vi "measVoltHzOffset.vi"() -> (1 "Error":bool)   [LabVIEW 2014]
uses:
  <vilib>/Platform/TimedLoop/XDataNode/timing_clust.ctl
  <vilib>/Platform/TimedLoop/XDataNode/nitl_modes.ctl
  <vilib>/Platform/TimedLoop/XDataNode/wakeup.ctl
  DAC/Code/FPGA SPI_Globals.vi
  <vilib>/rvi/Emulation/niFpgaSctlEmulationGetInTimedLoop.vi
  <vilib>/rvi/Emulation/niFpgaEmulationReportErrorSimple.vi
  <vilib>/rvi/Emulation/niFpgaGetClockAttributes.vi
  <vilib>/rvi/Emulation/niFpgaCriticalErrorInLSC.vi
  Sequencer/sequencerGlobVars.vi
  <vilib>/Platform/TimedLoop/XDataNode/XDataNode.xnode
  <vilib>/Platform/TimedLoop/XDataNode/XDNodeRunTimeDep.lvlib
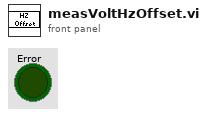
[diagram p1: front panel]
types:
  T1 = typedef "XDNodeRunTimeDep.lvlib/timing_clust.ctl" = cluster{"Expected End [f-1]":u64, "Actual End [f-1]":u64, "Finished Late? [f-1]":bool, "Expected End [i-1]":u64, "Actual End [i-1]":u64, "Finished Late? [i-1]":bool, "Expected Start [i]":u64, "Actual Start [i]":u64, "Expected Start [f]":u64, "Actual Start [f]":u64, "Source Name":string, "Structure Name":string, "Period":i64, "Deadline":i64, "Offset":i64, "Start":i64, "Priority":i32, "Timeout":i32, "Mode":T2, "Wakeup Reason":T3, "Error":errorcluster, "Source Type":string, "Secondary Source Type":string, "Global End Time":u64, "Global Start Time":u64, "Frame Duration":u64, "Iteration Duration":u64, "Assigned CPU":i32, "I/O Scan Engine Mode":u32}
  T2 = typedef "XDNodeRunTimeDep.lvlib/nitl_modes.ctl" = enum32{"No Change", "Process missed periods, maintain original phase", "Discard missed periods, maintain original phase", "Process missed periods, ignore original phase", "Discard missed periods, ignore original phase"}
  T3 = typedef "XDNodeRunTimeDep.lvlib/wakeup.ctl" = enum32{"Normal", "Aborted", "Asynchronous wakeup", "Timing source error", "Timed loop error", "Timeout"}
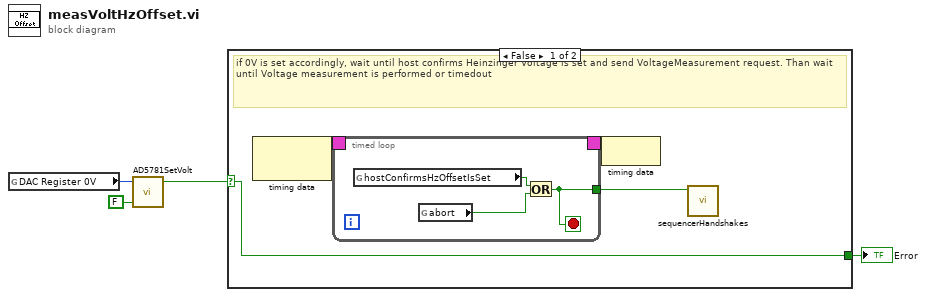
[diagram p0: block diagram]
diagram:
  n1 = global read "FPGA SPI_Globals.vi" "DAC Register 0V"() -> (w3:u32)
  n2 = call "AD5781SetVolt.vi"("Send"=FALSE, "SetVolt"=w3) -> ("timedOut"=w2:bool)  [unwired: 1 in, 2 out]
  n3 = case shown="False" w2 {
    selector: w2 -> [w5 w16]
    tunnel: [w5 w16] -> w1
    frame False {
      # "if 0V is set accordingly, wait until host confirms Heinzinger Voltage is set and send VoltageMeasurement request. Than wait until Voltage measurement is performed or timedout"
      n4 = node-c288() -> (w8:T1)  [unwired: 1 in]
      n5 = timed-loop {
        timing: w8 -> [_]
        timing-out: [_] -> w7
        tunnel: [w11] -> w6
        stop <- w11 stop-if-true
        n6 = global read "sequencerGlobVars.vi" "hostConfirmsHzOffsetIsSet"() -> (w9:bool)
        n7 = global read "sequencerGlobVars.vi" "abort"() -> (w10:bool)
        n8 = Or(x=w9, y=w10) -> (x .or. y?=w11:bool)
      }
      n9 = node-c288(w7) -> ()
      n10 = call "sequencerHandshakes.vi"("VoltOrScaler?"=w6) -> ()  [unwired: 11 in]
    }
    frame True {
    }
  }
  "Error" <- w1
